vi "UpdateSequenceIndicesTC.vi"(8 "error in (no error)":errorcluster, 11 "VMUI in":refnum<class "VMUI.lvclass">) -> (0 "error out":errorcluster, 3 "VMUI out":refnum<class "VMUI.lvclass">)   [LabVIEW 2013, in "VMUI.lvclass"]
uses:
  VMUI.lvclass
  <vilib>/Utility/miscctls.llb/LVRowAndColumnUnsignedTypeDef.ctl
  VariableManager/VariableManager.lvclass
  API/VariableManagerAPI.lvlib
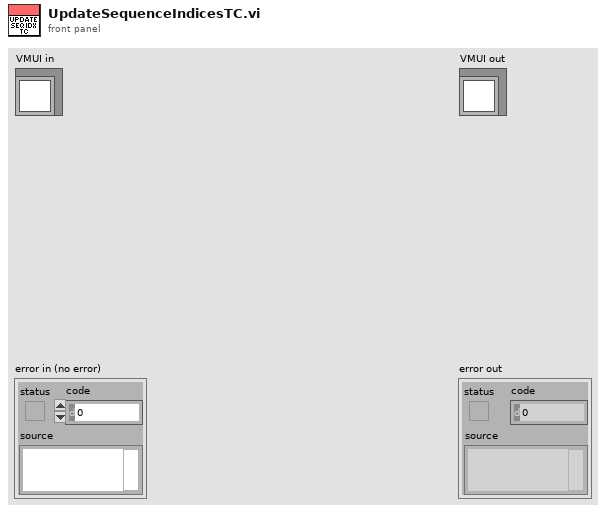
[diagram p1: front panel]
types:
  T1 = typedef "LVRowAndColumnUnsignedTypeDef.ctl" = cluster{"Row":u32, "Column":u32}
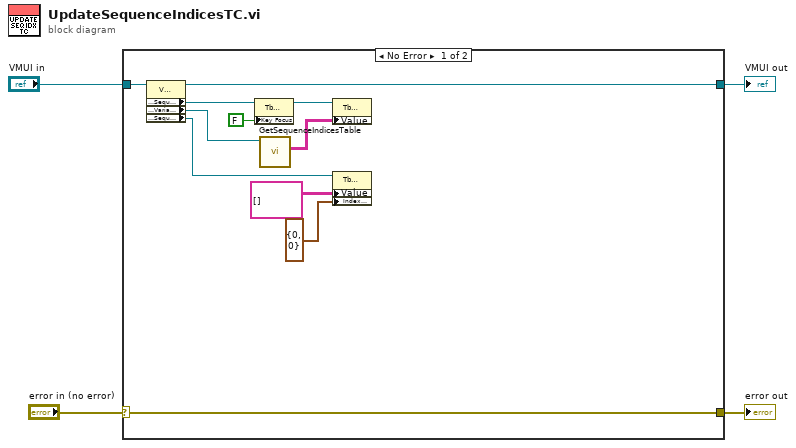
[diagram p0: block diagram]
diagram:
  n1 = case shown="No Error" "error in (no error)" {
    selector: "error in (no error)" -> [w14 w17]
    tunnel: [w14 w17] -> w3
    tunnel: [w13 w16] -> w1
    tunnel: "VMUI in" -> [w15 w16]
    frame No Error {
      n2 = property class="VMUI.lvclass"(reference=w15) -> (reference out=w13:refnum<class "VMUI.lvclass">, "Accessors:SequenceIndicesTCRef"=w9:refnum<vi>, "Accessors:VariableManagerRef"=w6:refnum<vi>, "Accessors:SequenceValuesTCRef"=w12:refnum<vi>)  [unwired: 1 in, 1 out]
      n3 = property class="Tbl (strict)"(reference=w9, "Key Focus"=FALSE) -> (reference out=w8:refnum<vi>)  [unwired: 1 in, 1 out]
      n4 = call "GetSequenceIndicesTable.vi"("VariableManagerRef in"=w6) -> ("SequenceIndicesTable"=w5:string[][])  [unwired: 8 in, 2 out]
      n5 = property class="Tbl (strict)"(reference=w8, "Value"=w5) -> ()  [unwired: 1 in, 2 out]
      n6 = property class="Tbl (strict)"(reference=w12, "Value"=string[][] [], "Index Values"=T1 {"Row"=0, "Column"=0}) -> ()  [unwired: 1 in, 2 out]
    }
    frame Error {
    }
  }
  "error out" <- w3
  "VMUI out" <- w1
